vi "re_sleep_lua.vi"(5 "LuaVIEW reference":T1) -> (15 "error out":errorcluster)   [LabVIEW 2012]
doc: "Puts a task to sleep. The task will be woken up when it receives a signal, message, or some custom event. The task can also be woken up after expiry of an optional timeout. When an event has occurred before going to sleep, the call will return immediately.\n\nBy testing for events after this function returns, tasks can quickly react without needing to poll. The timeout allows for a periodic wakeup call that has the task perform its standard chores.\n\nBefore going back to sleep, a task should test all the event types that it supports and handle them if they have occurred. The reason is that multiple events might occur before a task is woken from its sleep.\n\nIt might seem reasonable to reduce overhead by not testing events when a timed_out result of true is returned. This cannot be relied on. This function is based on \"Wait on Occurrence\", which, when called with an \"ignore previous\" input value of false very rarely keeps on returning \"timed out\" even though an occurrence was set. This bug is due to a race condition in LabVIEW <= 7.1 with a very tiny window of opportunity.\nParameters:\n[I32:timeout], optional timeout in milliseconds.\nResults:\nbool:timed_out, deprecated, do not rely on this result, see above.\nErrors:\nFunction must be called from a task context but was not."
uses:
  typedefs/t_LuaVIEW Reference.ctl
  typedefs/t_LuaVIEW Task State Methods.ctl
  subvis/private/LuaVIEW Push (boolean).vi
  subvis/private/LuaVIEW Pull (I32).vi
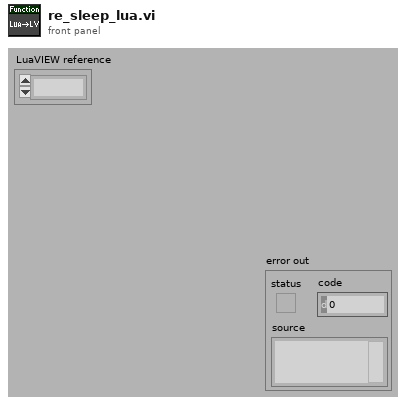
[diagram p1: front panel]
types:
  T1 = typedef "t_LuaVIEW Reference.ctl" = refnum<k1>
  T2 = typedef "t_LuaVIEW Task State Methods.ctl" = enum16{"cleanup", "set initial", "set mode", "set active mode", "set error", "get task info", "get script info", "set signal", "clear signal", "test handled", "test delegated", "test signal", "handle signal", "delegate signal", "allow signal", "disallow signal", "disallow all", "signals?", "delegated signals?", "protection++", "protection--", "protection=0", "message", "next message", "pop message", "message available?", "force stop", "set swap preps", "apply swap preps"}
  T3 = typedef "t_LuaVIEW Task State Pane.ctl" = refnum<vi>
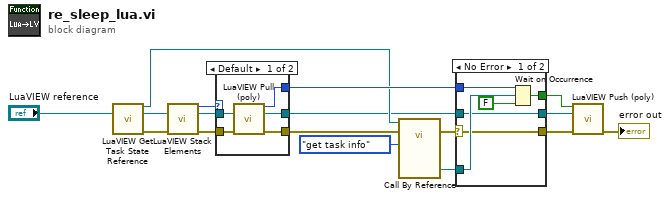
[diagram p0: block diagram]
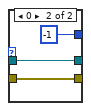
[diagram p3: hidden frame]
diagram:
  n1 = call "LuaVIEW Get Task State Reference.vi"("LuaVIEW reference in"="LuaVIEW reference") -> ("task state reference"=w7:T3, "LuaVIEW reference out"=w13:T1, "error out"=w12:errorcluster)  [unwired: 12 in]
  n2 = call "LuaVIEW Stack Elements.vi"("LuaVIEW reference in"=w13, "error in (no error)"=w12) -> ("elements"=w11:i32, "LuaVIEW reference out"=w10:T1, "error out"=w9:errorcluster)  [unwired: 11 in]
  n3 = case shown="Default" w11 {
    tunnel: w10 -> [w22 w25]
    tunnel: [w20 w25] -> w4
    tunnel: [w18 -1] -> w16
    tunnel: w9 -> [w21 w23]
    tunnel: [w19 w23] -> w8
    frame Default {
      n4 = call-poly "LuaVIEW Pull (poly).vi"("LuaVIEW reference in"=w22, "error in (no error)"=w21) -> ("I32"=w18:i32, "LuaVIEW reference out"=w20:T1, "error out"=w19:errorcluster)  [unwired: 11 in]
    }
    frame 0 {
    }
  }
  n5 = call-by-ref "?"(reference=w7, error in=w8, "method"=t_LuaVIEW_Task_State_Methods."get task info") -> (error out=w6:errorcluster, "wakeup occurrence"=w15:refnum<k4>)  [unwired: 10 in, 5 out]
  n6 = case shown="No Error" w6 {
    selector: w6 -> [w28 w33]
    tunnel: w16 -> [w31 _]
    tunnel: w15 -> [w29 _]
    tunnel: [w28 w33] -> w5
    tunnel: w4 -> [w26 w32]
    tunnel: [w26 w32] -> w3
    tunnel: [w27 _] -> w2
    frame No Error {
      n7 = Wait on Occurrence(1:FALSE ("ignore previous (T)"), 2:w29, 3:w31) -> (0:w27:bool)
    }
    frame Error {
    }
  }
  n8 = call-poly "LuaVIEW Push (poly).vi"("boolean"=w2, "LuaVIEW reference in"=w3, "error in (no error)"=w5) -> ("error out"=→"error out":errorcluster)  [unwired: 11 in, 1 out]
